vi "Linear Programming Middle.vi"(1 "C":dbl[](array[numeric]) format="%.2f", 2 "n-m*":u32[](array[numeric]), 3 "m*":u32[](array[numeric]), 4 "Table":dbl[][](array[numeric]) format="%.2f") -> (0 "Vector":dbl[](array[numeric]) format="%.2f")   [LabVIEW 2020, in "NI_Gmath.lvlib"]
uses:
  NI_Gmath.lvlib
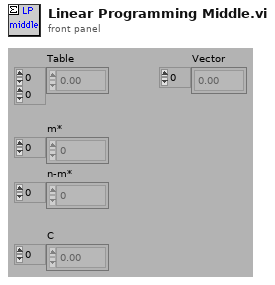
[diagram p1: front panel]
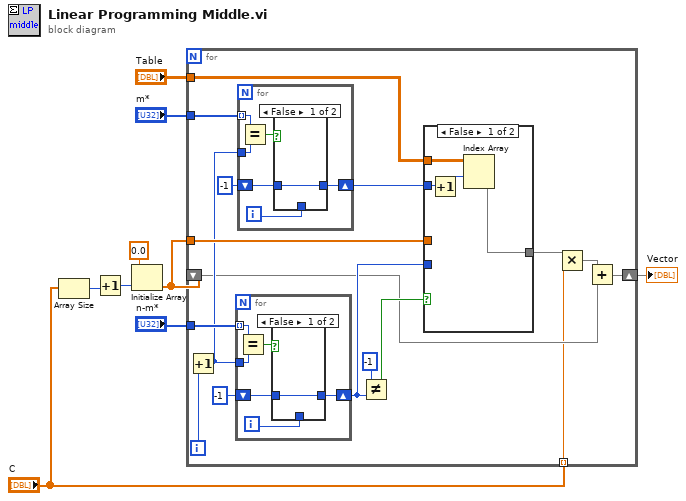
[diagram p0: block diagram]
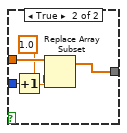
[diagram p2: hidden frame]
diagram:
  n1 = Array Size(array="C") -> (size(s)=w9:i32)
  n2 = Increment(x=w9) -> (x+1=w8:i32)
  n3 = Initialize Array(0.0, w8) -> (w6:dbl[])
  n4 = for {
    shift-right: [w13] -> w4
    shift-left: w6 -> [w14]
    tunnel: "n-m*" -> [w25]
    tunnel: "m*" -> [w23]
    tunnel: w6 -> [w20]
    tunnel: "Table" -> [w16]
    tunnel: "C" -> [w12] mode=indexing
    i -> [w26]
    n5 = Increment(x=w26) -> (x+1=w19:i32)
    n6 = for {
      tunnel: w19 -> [w49]
      tunnel: w25 -> [w48] mode=indexing
      shift-right: [w45] -> w18
      shift-left: -1 -> [w46]
      i -> [w44]
      n7 = Equal?(x=w48, y=w49) -> (x = y?=w47:bool)
      n8 = case shown="False" w47 {
        tunnel: w46 -> [w50 _]
        tunnel: [w50 w51] -> w45
        tunnel: w44 -> [_ w51]
        frame False {
        }
        frame True {
        }
      }
    }
    n9 = for {
      tunnel: w19 -> [w41]
      tunnel: w23 -> [w40] mode=indexing
      shift-right: [w37] -> w17
      shift-left: -1 -> [w38]
      i -> [w36]
      n10 = Equal?(x=w40, y=w41) -> (x = y?=w39:bool)
      n11 = case shown="False" w39 {
        tunnel: w38 -> [w42 _]
        tunnel: [w42 w43] -> w37
        tunnel: w36 -> [_ w43]
        frame False {
        }
        frame True {
        }
      }
    }
    n12 = Not Equal?(x=-1, y=w18) -> (x != y?=w15:bool)
    n13 = case shown="False" w15 {
      tunnel: w20 -> [_ w35]
      tunnel: w18 -> [_ w33]
      tunnel: w17 -> [w30 _]
      tunnel: w16 -> [w29 _]
      tunnel: [w28 w32] -> w10
      frame False {
        n14 = Increment(x=w30) -> (x+1=w27:i32)
        n15 = Index Array(array=w29, index (row)=w27) -> (element=w28:dbl[])  [unwired: 1 in]
      }
      frame True {
        n16 = Increment(x=w33) -> (x+1=w31:i32)
        n17 = Replace Array Subset(array=w35, new element=1.0, index=w31) -> (w32:dbl[])
      }
    }
    n18 = Multiply(x=w10, y=w12) -> (x*y=w11:dbl[])
    n19 = Add(x=w11, y=w14) -> (x+y=w13:dbl[])
  }
  "Vector" <- w4
